vi "Update channels.vi"(8 "error in (no error)":errorcluster, 11 "AOTF in":refnum<class "AOTF.lvclass">) -> (0 "error out":errorcluster, 3 "AOTF out":refnum<class "AOTF.lvclass">)   [LabVIEW 2012, in "AOTF.lvclass"]
uses:
  AOTF.lvclass
  AOTF.lvclass/AOTF.ctl
  <vilib>/DAQmx/write.llb/DAQmx Write (Digital 1D Bool 1Chan 1Samp).vi
  <vilib>/DAQmx/write.llb/DAQmx Write (Analog DBL 1Chan 1Samp).vi
  <vilib>/DAQmx/miscellaneous.llb/DAQmx Fill In Error Info.vi
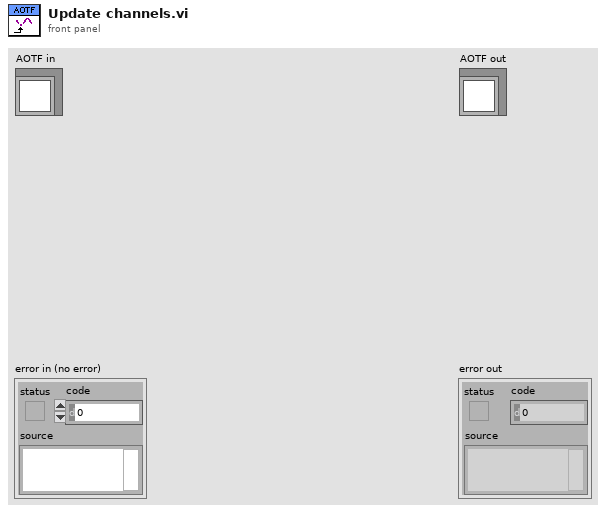
[diagram p1: front panel]
types:
  T1 = typedef "AOTF.lvclass/laser line ring.ctl" = u8
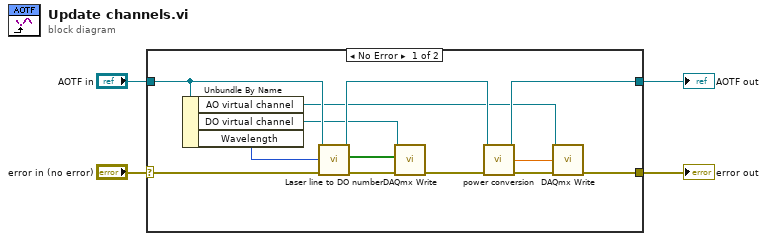
[diagram p0: block diagram]
diagram:
  n1 = case shown="No Error" "error in (no error)" {
    selector: "error in (no error)" -> [w12 w19]
    tunnel: [w17 w19] -> w3
    tunnel: [w16 w18] -> w1
    tunnel: "AOTF in" -> [w10 w18]
    frame No Error {
      n2 = Unbundle By Name(w10) -> ("AO virtual channel"=w6:refnum<k21>, "DO virtual channel"=w7:refnum<k21>, "Wavelength"=w8:T1)
      n3 = call-dynamic "Laser line to DO number.vi"("error in (no error)"=w12, "Wavelength"=w8, "AOTF in"=w10) -> ("error out"=w11:errorcluster, "DO number"=w5:bool[], "AOTF out"=w9:refnum<class "AOTF.lvclass">)  [unwired: 6 in]
      n4 = call-poly <vilib>:"DAQmx Write.vi"("task/channels in"=w7, "data"=w5, "error in"=w11) -> ("error out"=w15:errorcluster)  [unwired: 10 in, 2 out]
      n5 = call-dynamic "power conversion.vi"("error in (no error)"=w15, "AOTF in"=w9) -> ("error out"=w14:errorcluster, "Power voltage out"=w13:dbl, "AOTF out"=w16:refnum<class "AOTF.lvclass">)  [unwired: 7 in]
      n6 = call-poly <vilib>:"DAQmx Write.vi"("task/channels in"=w6, "data"=w13, "error in"=w14) -> ("error out"=w17:errorcluster)  [unwired: 10 in, 2 out]
    }
    frame Error {
    }
  }
  "error out" <- w3
  "AOTF out" <- w1
